vi "test VIT Verify MultiCombos.vi"(8 "error in":errorcluster, 11 "Testing Approval Tests in":refnum<class "VITester Extension Tests.lvclass">) -> (0 "error out":errorcluster, 3 "Testing Approval Tests out":refnum<class "VITester Extension Tests.lvclass">)   [LabVIEW 2026, in "VITester Extension Tests.lvclass"]
uses:
  VITester Extension Tests.lvclass
  f2b1d098-7b1d-4c0a-8a43-3da18094a121.vi
  85b95d5f-c096-4ded-91f8-32f3feefbab9.vi
  f9c159a5-2828-4b5e-be94-bc98101363dc.vi
  VITester Extension Tests.lvclass/VITester Extension Tests.ctl
  Source/Extensions/VITester.Extension/VITester.Extension.lvlib
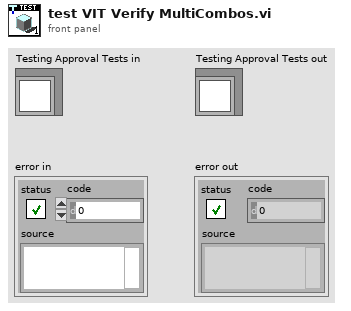
[diagram p1: front panel]
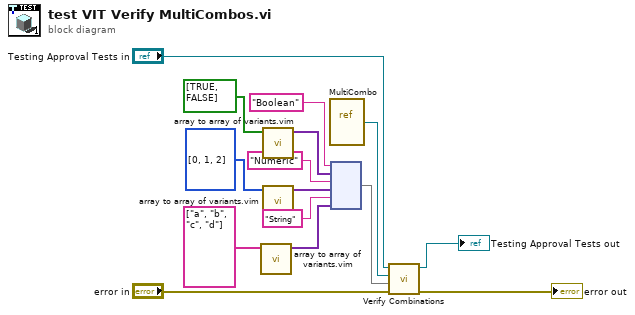
[diagram p0: block diagram]
diagram:
  n1 = call "array to array of variants.vim"("Array in"=string[] ["a", "b", "c", "d"]) -> ("Array out"=w6:variant[])  [unwired: 10 in]
  n2 = call "array to array of variants.vim"("Array in"=bool[] [TRUE, FALSE]) -> ("Array out"=w9:variant[])  [unwired: 10 in]
  n3 = call "array to array of variants.vim"("Array in"=i32[] [0, 1, 2]) -> ("Array out"=w7:variant[])  [unwired: 10 in]
  n4 = vi-ref "MultiCombo.vi"() -> (w3:refnum<vi>)
  n5 = node ("Build Map")("Boolean" ("key"), w9, "Numeric" ("key"), w7, "String" ("key"), w6) -> (w2:map{string, variant[]})
  n6 = call "Verify Combinations.vi"("error in"="error in", "ctl label -> value var[]"=w2, "VI Refnum"=w3, "TestCase in"="Testing Approval Tests in") -> ("error out"=→"error out":errorcluster, "TestCase out"=→"Testing Approval Tests out":refnum<class "VITester Extension Tests.lvclass">)  [unwired: 6 in]
